vi "Initialize.vi"(8 "error in (no error)":errorcluster, 10 "Parameters in":refnum<class "Abstract Init Parameters.lvclass">[](array[class]), 11 "Abstract Producer in":refnum<class "Abstract Producer.lvclass">) -> (0 "error out":errorcluster, 3 "Abstract Producer out":refnum<class "Abstract Producer.lvclass">)   [LabVIEW 2017, in "Messaging.lvlib" / "Abstract Producer.lvclass"]
uses:
  Abstract Producer.lvclass
  Parameters/Abstract Init Parameters/Abstract Init Parameters.lvclass
  Consumer Information.ctl
  Message Queue/Abstract Message Queue/Abstract Message Queue.lvclass
  Abstract Producer.lvclass/Abstract Producer.ctl
  Messaging.lvlib
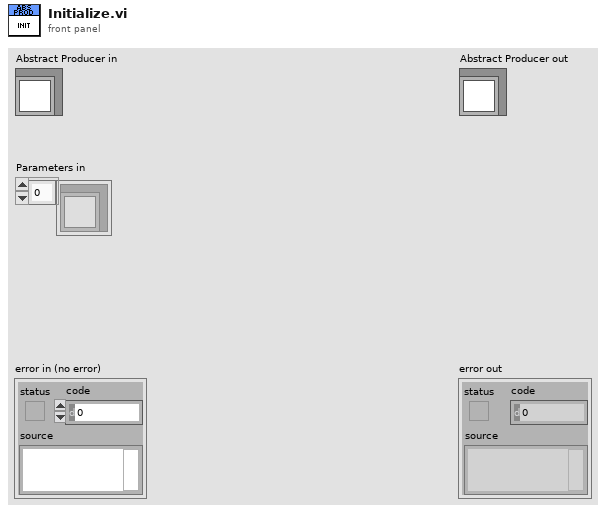
[diagram p1: front panel]
types:
  T1 = typedef "Messaging.lvlib/Abstract Producer.lvclass/Consumer Information.ctl" = cluster{"Name":string, "Request Queue":refnum<class "Abstract Message Queue.lvclass">, "Response Queue":refnum<class "Abstract Message Queue.lvclass">}
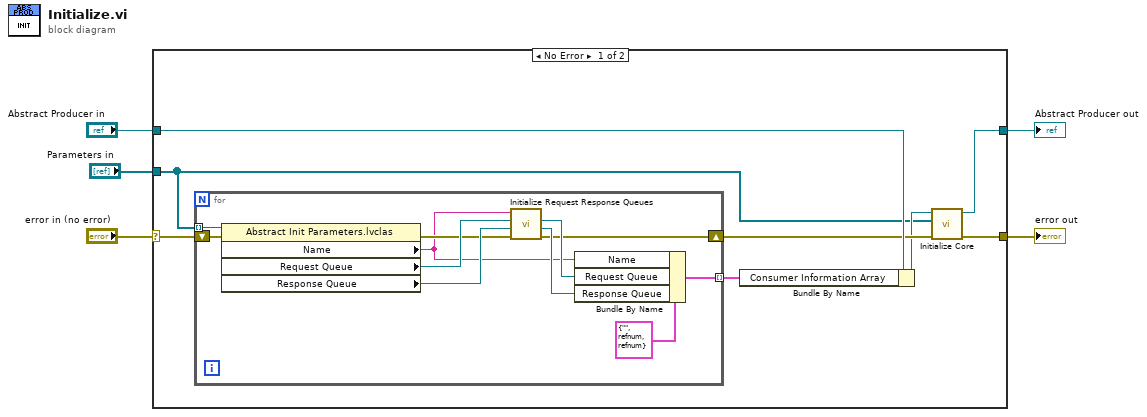
[diagram p0: block diagram]
diagram:
  n1 = case shown="No Error" "error in (no error)" {
    selector: "error in (no error)" -> [w13 w26]
    tunnel: [w9 w26] -> w4
    tunnel: [w7 w25] -> w2
    tunnel: "Abstract Producer in" -> [w11 w25]
    tunnel: "Parameters in" -> [w6 _]
    frame No Error {
      n2 = for {
        tunnel: w6 -> [w24] mode=indexing
        shift-right: [w14] -> w10
        shift-left: w13 -> [w23]
        tunnel: [w15] -> w12 mode=indexing
        n3 = property class="Abstract Init Parameters.lvclas"(reference=w24, error in=w23) -> (error out=w20:errorcluster, "Name"=w16:string, "Request Queue"=w22:refnum<class "Abstract Message Queue.lvclass">, "Response Queue"=w21:refnum<class "Abstract Message Queue.lvclass">)  [unwired: 1 out]
        n4 = call "Initialize Request Response Queues.vi"("error in (no error)"=w20, "Response Queue in"=w21, "Request Queue in"=w22, "Name"=w16) -> ("error out"=w14:errorcluster, "Response Queue out"=w17:refnum<class "Abstract Message Queue.lvclass">, "Request Queue out"=w18:refnum<class "Abstract Message Queue.lvclass">)  [unwired: 5 in]
        n5 = Bundle By Name(cluster=T1 {"Name"="", "Request Queue"=refnum, "Response Queue"=refnum} ("Consumer Information"), "Name"=w16, "Request Queue"=w18, "Response Queue"=w17) -> (w15:T1)
      }
      n6 = Bundle By Name(cluster=w11, "Consumer Information Array"=w12) -> (w8:refnum<class "Abstract Producer.lvclass">)
      n7 = call-dynamic "Initialize Core.vi"("error in (no error)"=w10, "Parameters"=w6, "Abstract Producer in"=w8) -> ("error out"=w9:errorcluster, "Abstract Producer out"=w7:refnum<class "Abstract Producer.lvclass">)  [unwired: 7 in]
    }
    frame Error {
    }
  }
  "error out" <- w4
  "Abstract Producer out" <- w2
